vi "Connect Error Wires.vi"(0 "Node in":refnum<vi>, 5 "New Object Ref":refnum<vi>, 9 "String":string, 11 "error in (no error)":errorcluster) -> (15 "error out":errorcluster)   [LabVIEW 2021, in "Converter.lvlib"]
uses:
  Converter.lvlib
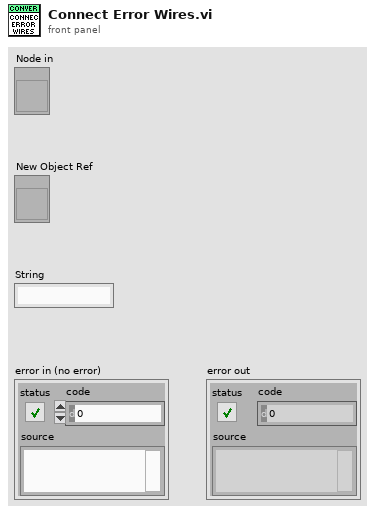
[diagram p1: front panel]
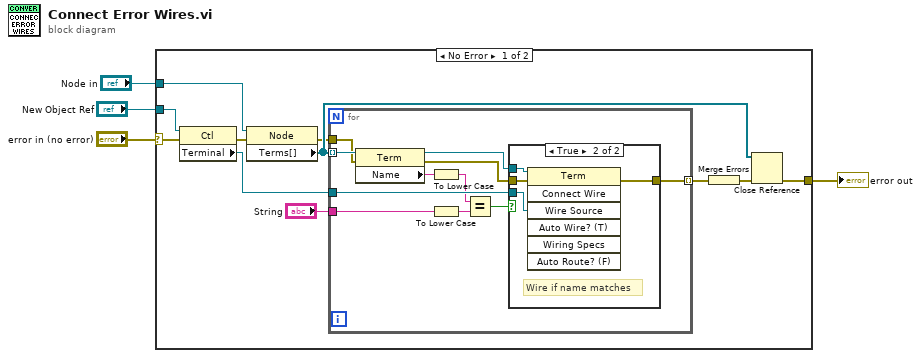
[diagram p0: block diagram]
diagram:
  n1 = case shown="No Error" "error in (no error)" {
    selector: "error in (no error)" -> [w14 w32]
    tunnel: "New Object Ref" -> [w12 _]
    tunnel: [w10 w32] -> w2
    tunnel: "Node in" -> [w5 _]
    frame No Error {
      n2 = property class="Ctl"(reference=w12, error in=w14) -> (error out=w13:errorcluster, "Terminal"=w15:refnum<vi>)  [unwired: 1 out]
      n3 = property class="Node"(reference=w5, error in=w13) -> (error out=w6:errorcluster, "Terms[]"=w11:refnum<vi>[])  [unwired: 1 out]
      n4 = for {
        tunnel: w11 -> [w26] mode=indexing
        tunnel: w6 -> [w25]
        tunnel: "String" -> [w23]
        tunnel: [w19] -> w8 mode=indexing
        tunnel: w15 -> [w18]
        n5 = property class="Term"(reference=w26, error in=w25) -> (reference out=w20:refnum<vi>, error out=w21:errorcluster, "Name"=w24:string)
        n6 = To Lower Case(string=w24) -> (all lower case string=w17:string)
        n7 = To Lower Case(string=w23) -> (all lower case string=w16:string)
        n8 = Equal?(x=w17, y=w16) -> (x = y?=w22:bool)
        n9 = case shown="True" w22 {
          tunnel: w21 -> [w27 w31]
          tunnel: w20 -> [_ w30]
          tunnel: [w27 w29] -> w19
          tunnel: w18 -> [_ w28]
          frame False {
          }
          frame True {
            # "Wire if name matches"
            n10 = invoke class="Term" method="Connect Wire"(reference=w30, error in=w31, "Wire Source"=w28) -> (error out=w29:errorcluster)  [unwired: 4 in, 6 out]
          }
        }
      }
      n11 = Merge Errors(w8) -> (w9:errorcluster)
      n12 = Close Reference(reference=w11, error in (no error)=w9) -> (error out=w10:errorcluster)
    }
    frame Error {
    }
  }
  "error out" <- w2
